vi "Initialize.vi"(8 "error in (no error)":errorcluster, 9 "Reset (True)":bool=TRUE, 10 "ID Query (True)":bool=TRUE, 11 "VISA resource name":refnum<visa-resource-name>) -> (0 "error out":errorcluster, 3 "VISA resource name out":refnum<visa-resource-name>)   [LabVIEW 2015, in "RIGOL DP800 Series.lvlib"]
doc: "Establishes communication with the instrument and optionally performs an instrument identification query and/or an instrument reset. It also places the instrument in a default state needed for other instrument driver operations. Therefore, call this VI before calling other instrument driver VIs for this instrument. Generally, you need to call the Initialize VI only once at the beginning of an application."
uses:
  <instrlib>/RIGOL DP800 Series/RIGOL DP800 Series.lvlib
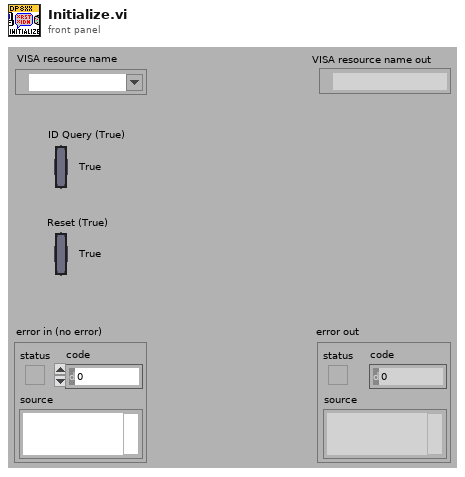
[diagram p1: front panel]
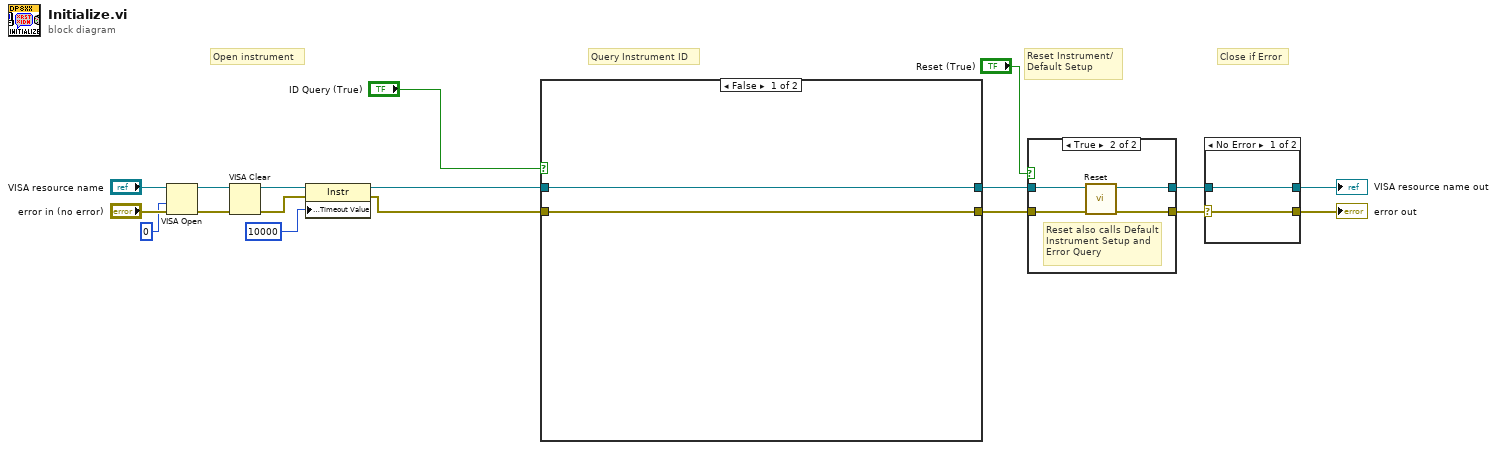
[diagram p0: block diagram]
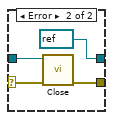
[diagram p2: hidden frame]
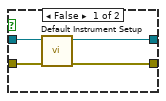
[diagram p3: hidden frame]
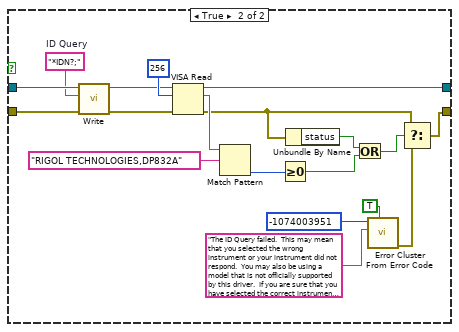
[diagram p4: hidden frame]
diagram:
  # "Close if Error"
  # "Query Instrument ID"
  # "Reset Instrument/\nDefault Setup"
  # "Open instrument"
  n1 = VISA Open(access mode=u32 0, error in (no error)="error in (no error)", VISA resource name="VISA resource name") -> (VISA resource name=w10:refnum<visa-resource-name>, error out=w9:errorcluster)  [unwired: 2 out]
  n2 = VISA Clear(VISA resource name=w10, error in (no error)=w9) -> (VISA resource name out=w8:refnum<visa-resource-name>, error out=w7:errorcluster)
  n3 = property class="Instr"(reference=w8, error in=w7, "General Settings:Timeout Value"=u32 10000) -> (reference out=w2:refnum<visa-resource-name>, error out=w1:errorcluster)
  n4 = case shown="False" "ID Query (True)" {
    tunnel: [w19 w39] -> w17
    tunnel: [w20 w38] -> w18
    tunnel: w2 -> [w20 w22]
    tunnel: w1 -> [w19 w23]
    frame False {
    }
    frame True {
      w21 = "*IDN?;"  # ID Query
      n5 = call <instrlib>:"Write.vi"("error in (no error)"=w23, "Write Buffer (\"\")"=w21, "VISA resource name"=w22) -> ("error out"=w24:errorcluster, "VISA resource name out"=w25:refnum<visa-resource-name>)  [unwired: 7 in]
      n6 = VISA Read(VISA resource name=w25, byte count=u32 256, error in (no error)=w24) -> (VISA resource name out=w38:refnum<visa-resource-name>, read buffer=w37:string, error out=w29:errorcluster)  [unwired: 1 out]
      n7 = Match Pattern(string=w37, regular expression="RIGOL TECHNOLOGIES,DP832A") -> (offset past match=w30:i32)  [unwired: 4 out]
      n8 = Greater Or Equal To 0?(x=w30) -> (x >= 0?=w27:bool)
      n9 = Unbundle By Name(w29) -> ("status"=w28:bool)
      n10 = Or(x=w28, y=w27) -> (x .or. y?=w26:bool)
      n11 = call <vilib>:"Error Cluster From Error Code.vi"("show call chain? (False)"=TRUE, "error message (\"\")"="The ID Query failed.  This may mean that you selected the wrong instrument or your instrument did not respond.  You may also be using a model that is not officially supported by this driver.  If you are sure that you have selected the correct instrument and it is responding, try disabling the ID Query." ("Source (VI Name)"), "error code (0)"=-1074003951 ("Code")) -> ("error out"=w34:errorcluster)  [unwired: 1 in, 5 out]
      n12 = Select(t=w29, s=w26, f=w34) -> (s? t:f=w39:errorcluster)
    }
  }
  n13 = case shown="True" "Reset (True)" {
    tunnel: w17 -> [w42 w44]
    tunnel: [w40 w47] -> w3
    tunnel: w18 -> [w43 w45]
    tunnel: [w41 w46] -> w4
    frame False {
      n14 = call <instrlib>:"Default Instrument Setup.vi"("error in (no error)"=w42, "VISA resource name"=w43) -> ("error out"=w40:errorcluster, "VISA resource name out"=w41:refnum<visa-resource-name>)  [unwired: 8 out]
    }
    frame True {
      # "Reset also calls Default Instrument Setup and Error Query"
      n15 = call <instrlib>:"Reset.vi"("error in (no error)"=w44, "VISA resource name"=w45) -> ("error out"=w47:errorcluster, "VISA resource name out"=w46:refnum<visa-resource-name>)  [unwired: 8 out]
    }
  }
  n16 = case shown="No Error" w3 {
    selector: w3 -> [w48 w51]
    tunnel: w4 -> [w49 w52]
    tunnel: [w49 refnum<visa-resource-name> refnum ("VISA resource name out")] -> w6
    tunnel: [w48 w53] -> w5
    frame No Error {
    }
    frame Error {
      n17 = call <instrlib>:"Close.vi"("error in (no error)"=w51, "VISA resource name"=w52) -> ("error out"=w53:errorcluster)  [unwired: 9 out]
    }
  }
  "VISA resource name out" <- w6
  "error out" <- w5
